vi "900x 9870 Interrupt Write (Sub).vi"(8 "error in":errorcluster, 10 "Data":string, 11 "FPGA In":T1) -> (0 "error out":errorcluster, 1 "Byte Count":u32, 3 "FPGA Out":T1, 4 "Timed Out":bool, 6 "FPGA Error":errorcluster)   [LabVIEW 2012]
uses:
  900x INT FPGA Reference.ctl
  FPGA Function.ctl
  <vilib>/Utility/error.llb/Error Cluster From Error Code.vi
  <vilib>/rvi/errors/niLvFpgaAdjustHostInterfaceError.vi
  <vilib>/rvi/interface/nirviReadWriteControl/nirviReadWriteControl.xnode
  FPGA Bitfiles/NI-987xSerialLoo_FPGATarget3_9870InterfaceInt_BB93BC1A.lvbitx
  Program Files (x86)/National Instruments/LabVIEW 2012/examples/CompactRIO/Module Specific/NI 987x/Serial Loopback/VIs/9870 Interface Interrupt (FPGA).vi
  <vilib>/rvi/interface/nirviMethod/nirviMethod.xnode
  NiFpgaLv.dll
  <vilib>/FPGAPlugInAG/cRIO-9101/niLvFpga_AcknowledgeIrq_cRIO-9101.vi
  <vilib>/rvi/interface/nirviMethod/StockFPGA_InlinedMethodWaitForSingleIRQ.vi
  <vilib>/FPGAPlugInAG/cRIO-9101/niLvFpga_WaitOnIrq_cRIO-9101.vi
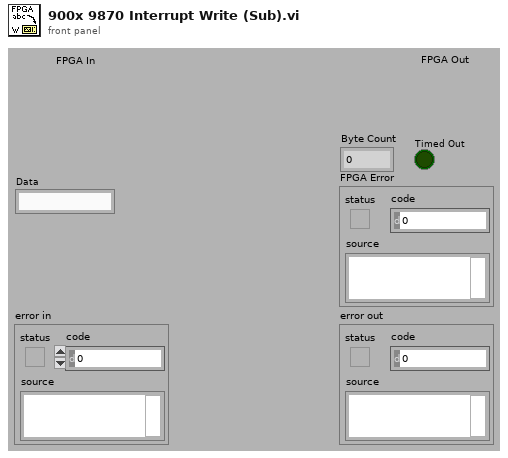
[diagram p1: front panel]
types:
  T1 = typedef "900x INT FPGA Reference.ctl" = refnum<k20>
  T2 = typedef "FPGA Function.ctl" = enum16{"Do Nothing", "Write", "Read"}
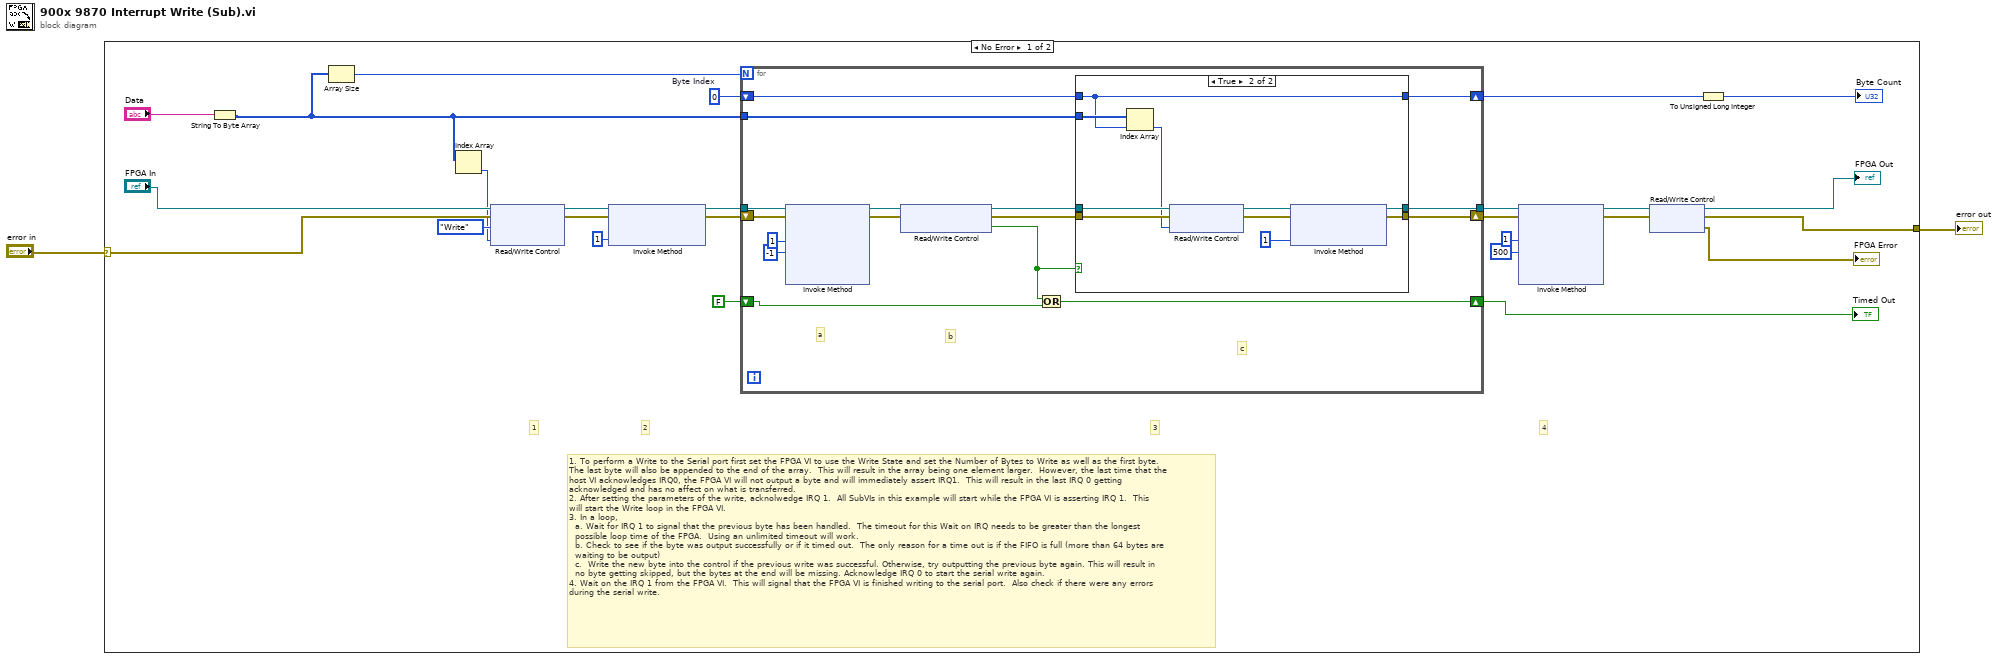
[diagram p0: block diagram]
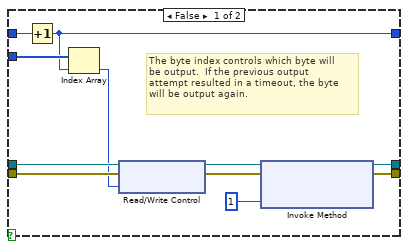
[diagram p2: hidden frame]
diagram:
  n1 = case shown="No Error" "error in" {
    selector: "error in" -> [w9 w66]
    tunnel: [w5 w66] -> w1
    frame No Error {
      w19 = 0  # Byte Index
      # "4"
      # "3"
      # "2"
      # "1"
      # "1. To perform a Write to the Serial port first set the FPGA VI to use the Write State and set the Number of Bytes to Write as well as the first byte.\nThe last byte will also be appended to the end of the array.  This will result in the array being one element larger.  However, the last time that the\nhost VI acknowledges IRQ0, the FPGA VI will not output a byte and will immediately assert IRQ1.  This will result in the last IRQ 0 getting \nacknowledged and has no affect on what is transferred.\n2. After setting the parameters of the write, acknolwedge IRQ 1.  All SubVIs in this example will start while the FPGA VI is asserting IRQ 1.  This \nwill start the Write loop in the FPGA VI.\n3. In a loop, \n  a. Wait for IRQ 1 to signal that the previous byte has been handled.  The timeout for this Wait on IRQ needs to be greater than the longest \n  possible loop time of the FPGA.  Using an unlimited timeout will work.\n  b. Check to see if the byte was output successfully or if it timed out.  The only reason for a time out is if the FIFO is full (more than 64 bytes are \n  waiting to be output)\n  c.  Write the new byte into the control if the previous write was successful. Otherwise, try outputting the previous byte again. This will result in \n  no byte getting skipped, but the bytes at the end will be missing. Acknowledge IRQ 0 to start the serial write again.\n4. Wait on the IRQ 1 from the FPGA VI.  This will signal that the FPGA VI is finished writing to the serial port.  Also check if there were any errors\nduring the serial write."
      n2 = String To Byte Array(string="Data") -> (unsigned byte array=w4:u8[])
      n3 = Array Size(array=w4) -> (size(s)=w16:i32)
      n4 = Index Array(array=w4) -> (element=w3:u8)  [unwired: 1 in]
      n5 = xnode "Read/Write Control"("FPGA VI Reference In"="FPGA In", "error in"=w9, "Op Control"=FPGA_Function."Write", "Byte to Write"=w3) -> ("FPGA VI Reference Out"=w21:T1, "error out"=w17:errorcluster)
      n6 = xnode "Invoke Method"("FPGA VI Reference In"=w21, "error in"=w17, "IRQ Number(s)"=1) -> ("FPGA VI Reference Out"=w23:T1, "error out"=w18:errorcluster)
      n7 = for {
        N: w16 -> [_]
        tunnel: w23 -> [w43]
        tunnel: [w44] -> w25
        shift-right: [w42] -> w24
        shift-left: w18 -> [w41]
        shift-right: [w32] -> w28
        shift-left: FALSE ("Timed Out") -> [w33]
        shift-right: [w39] -> w8
        shift-left: w19 -> [w34]
        tunnel: w4 -> [w30]
        # "c"
        # "b"
        # "a"
        n8 = xnode "Invoke Method"("FPGA VI Reference In"=w43, "error in"=w41, "IRQ Number(s)"=1, "Timeout (ms)"=-1) -> ("FPGA VI Reference Out"=w38:T1, "error out"=w35:errorcluster)  [unwired: 2 out]
        n9 = xnode "Read/Write Control"("FPGA VI Reference In"=w38, "error in"=w35) -> ("FPGA VI Reference Out"=w37:T1, "error out"=w36:errorcluster, "Timed Out Write"=w31:bool)
        n10 = Or(x=w31, y=w33) -> (x .or. y?=w32:bool)
        n11 = case shown="True" w31 {
          tunnel: [w50 w60] -> w44
          tunnel: [w49 w59] -> w42
          tunnel: w37 -> [w52 w62]
          tunnel: w36 -> [w51 w61]
          tunnel: w34 -> [w46 w56]
          tunnel: [w45 w56] -> w39
          tunnel: w30 -> [w48 w58]
          frame False {
            # "The byte index controls which byte will \nbe output.  If the previous output \nattempt resulted in a timeout, the byte\nwill be output again."
            n12 = Increment(x=w46) -> (x+1=w45:i32)
            n13 = Index Array(array=w48, index=w45) -> (element=w47:u8)
            n14 = xnode "Read/Write Control"("FPGA VI Reference In"=w52, "error in"=w51, "Byte to Write"=w47) -> ("FPGA VI Reference Out"=w53:T1, "error out"=w54:errorcluster)
            n15 = xnode "Invoke Method"("FPGA VI Reference In"=w53, "error in"=w54, "IRQ Number(s)"=1) -> ("FPGA VI Reference Out"=w50:T1, "error out"=w49:errorcluster)
          }
          frame True {
            n16 = Index Array(array=w58, index=w56) -> (element=w57:u8)
            n17 = xnode "Read/Write Control"("FPGA VI Reference In"=w62, "error in"=w61, "Byte to Write"=w57) -> ("FPGA VI Reference Out"=w63:T1, "error out"=w64:errorcluster)
            n18 = xnode "Invoke Method"("FPGA VI Reference In"=w63, "error in"=w64, "IRQ Number(s)"=1) -> ("FPGA VI Reference Out"=w60:T1, "error out"=w59:errorcluster)
          }
        }
      }
      "Timed Out" <- w28
      n19 = xnode "Invoke Method"("FPGA VI Reference In"=w25, "error in"=w24, "IRQ Number(s)"=1, "Timeout (ms)"=500) -> ("FPGA VI Reference Out"=w12:T1, "error out"=w11:errorcluster)  [unwired: 2 out]
      n20 = xnode "Read/Write Control"("FPGA VI Reference In"=w12, "error in"=w11) -> ("FPGA VI Reference Out"=→"FPGA Out":T1, "error out"=w5:errorcluster, "error out"=→"FPGA Error":errorcluster)
      n21 = To Unsigned Long Integer(number=w8) -> (unsigned 32bit integer=→"Byte Count":u32)
    }
    frame Error {
    }
  }
  "error out" <- w1
